vi "Measure Digital Pulse PtByPt.vi"(4 "stop (F)":bool, 6 "timeout (units)":i32=720000, 7 "cycles to filter (0)":u16, 8 "inverted pulse (F)":bool, 9 "start time (units)":u32, 10 "current time (units)":u32, 11 "FPGA digital input":refnum<k21>="Port0/DIO0") -> (1 "timed out?":bool, 2 "stopped?":bool, 3 "pulse width (units)":u32)   [LabVIEW 2017, in "NI_Robotics_FPGA Utilities.lvlib"]
uses:
  <vilib>/robotics/Utilities/FPGA Utilities/NI_Robotics_FPGA Utilities.lvlib
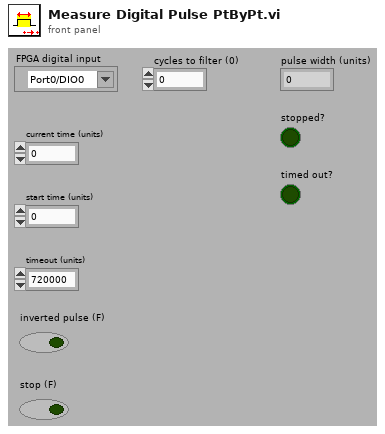
[diagram p1: front panel]
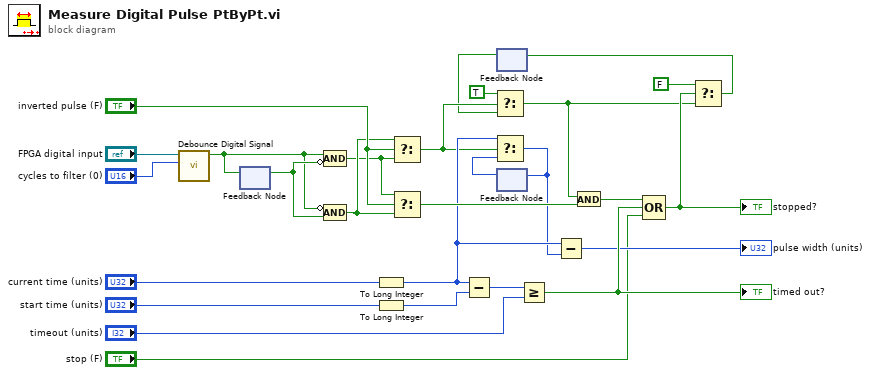
[diagram p0: block diagram]
diagram:
  n1 = call <vilib>:"Debounce Digital Signal.vi"("cycles to filter (0)"="cycles to filter (0)", "FPGA digital input"="FPGA digital input") -> ("filtered output"=w3:bool)  [unwired: 9 in]
  n2 = feedback #1() -> (w27:bool)  [unwired: 1 out]
  n3 = feedback-in #1(w3) -> ()
  n4 = Compound Arithmetic op=AND(w3, invert w27) -> (w23:bool)
  n5 = Compound Arithmetic op=AND(invert w3, w27) -> (w24:bool)
  n6 = To Long Integer(number="current time (units)") -> (32bit integer=w11:i32)
  n7 = To Long Integer(number="start time (units)") -> (32bit integer=w15:i32)
  n8 = Select(t=w24, s="inverted pulse (F)", f=w23) -> (s? t:f=w8:bool)
  n9 = Select(t=w23, s="inverted pulse (F)", f=w24) -> (s? t:f=w22:bool)
  n10 = Subtract(x=w11, y=w15) -> (x-y=w18:i32)
  n11 = feedback #2() -> (w5:bool)  [unwired: 1 in]
  n12 = Select(t=TRUE, s=w8, f=w5) -> (s? t:f=w6:bool)
  n13 = feedback #3() -> (w9:i32)  [unwired: 1 in]
  n14 = Select(t=w11, s=w8, f=w9) -> (s? t:f=w10:i32)
  n15 = feedback-in #3(w10) -> ()
  n16 = Greater Or Equal?(x=w18, y="timeout (units)") -> (x >= y?=w26:bool)
  "timed out?" <- w26
  n17 = Subtract(x=w11, y=w10) -> (x-y=→"pulse width (units)":i32)
  n18 = And(x=w6, y=w22) -> (x .and. y?=w20:bool)
  n19 = Compound Arithmetic op=OR(w20, w26, "stop (F)") -> (w14:bool)
  "stopped?" <- w14
  n20 = Select(t=FALSE, s=w14, f=w6) -> (s? t:f=w13:bool)
  n21 = feedback-in #2(w13) -> ()
